vi "callback_right button.vi"(4 "User Parameter":refnum<vi>, 6 "CtlRef":refnum<vi>, 7 "Event Common Data":cluster{"Source":T1, "Type":T2, "Time":u32} {"Source" items=["LabVIEW UI"=0, "ActiveX"=1, "User Event"=25]}) -> ()   [LabVIEW 2009]
uses:
  <vilib>/event_ctls.llb/eventsource.ctl
  <vilib>/event_ctls.llb/lveventtype.ctl
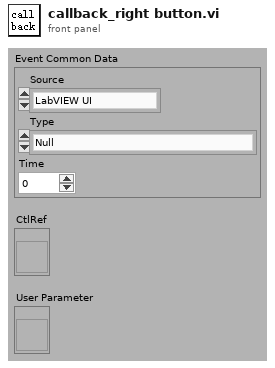
[diagram p1: front panel]
types:
  T1 = typedef "eventsource.ctl" = u32
  T2 = typedef "lveventtype.ctl" = enum32{"Null", "Timeout", "App Instance Close", "App Instance Close?", "Cell Edit", "Cell Edit?", "Cursor Grab", "Cursor Grab?", "Cursor Move", "Cursor Release", "Data Change", "Direction Change", "Display State Change", "Drag Ended", "Drag Enter", "Drag Leave", "Drag Over", "Drag Source Update", "Drag Starting", "Drag Starting?", "Drop", "Exec State Change", "Key Down", "Key Down?", "Key Repeat", "Key Repeat?", "Key Up", "Listbox Double Click", "Menu Activation?", "Menu Selection (App)", "Menu Selection? (App)", "Menu Selection (User)", "Mouse Down", "Mouse Down?", "Mouse Enter", "Mouse Leave", "Mouse Move", "Mouse Up", "NI Security User Change (App)", "Pane Size", "Panel Close", "Panel Close?", "Panel Resize", "Plot Attribute Change", "Scale Range Change", "Shortcut Menu Activation?", "Shortcut Menu Selection (App)", "Shortcut Menu Selection? (App)", "Shortcut Menu Selection (User)", "Tree Double Click", "Tree Drag", "Tree Drag?", "Tree Drop", "Tree Drop?", "Tree Item Close", "Tree Item Close?", "Tree Item Open", "Tree Item Open?", "Value Change"}
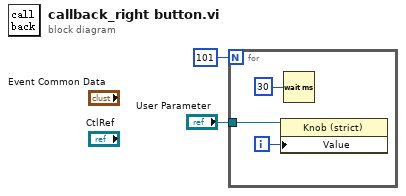
[diagram p0: block diagram]
diagram:
  n1 = for {
    N: 101 -> [_]
    tunnel: "User Parameter" -> [w5]
    i -> [w4]
    n2 = property class="Knob (strict)"(reference=w5, "Value"=w4) -> ()  [unwired: 1 in, 2 out]
    n3 = Wait (ms)(milliseconds to wait=u32 30) -> ()  [unwired: 1 out]
  }
